vi "Define_Size_of_Array_Connected_Tracks-1.vi"(3 "[IN] Size of Longest Array\nbetween Subtracks (0,0)":i32, 4 "[IN] Indexes for Jumps":i32[](array[numeric]), 5 "[IN] Original Array Size":i32, 6 "[IN] Dot Statuses":i16[][](array[numeric])) -> (1 "[OUT] # of Eleme\nnts in new Track":i32)   [LabVIEW 2013]
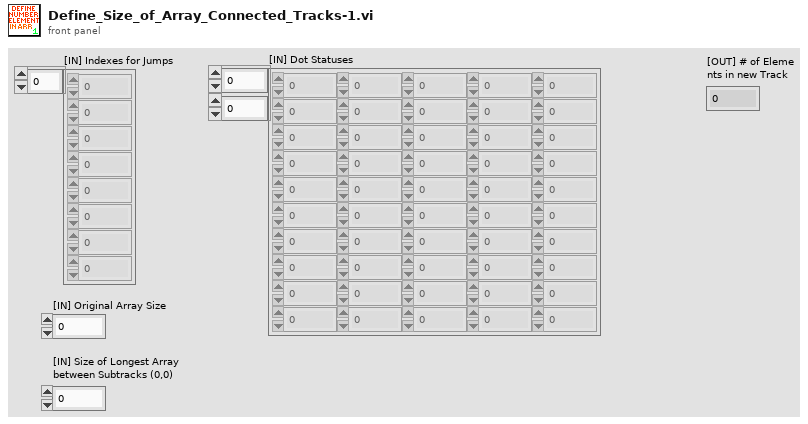
[diagram p1: front panel]
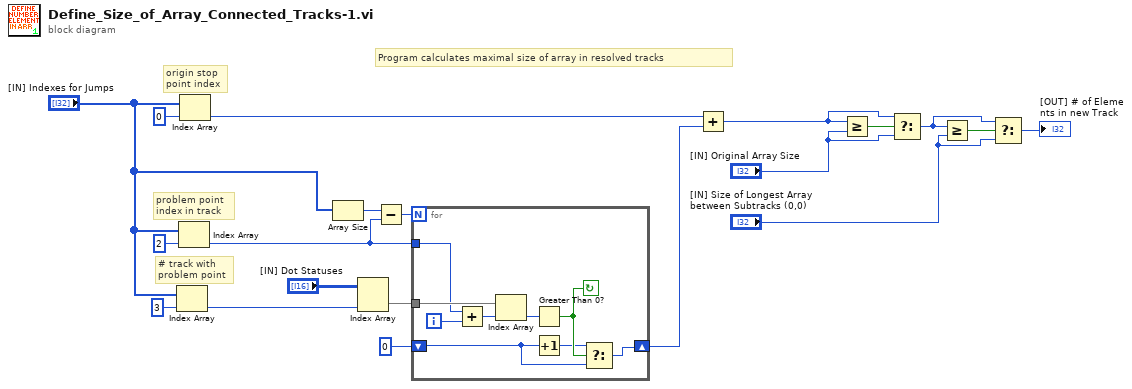
[diagram p0: block diagram]
diagram:
  # "Program calculates maximal size of array in resolved tracks"
  # "# track with \nproblem point"
  # "problem point \nindex in track"
  # "origin stop \npoint index"
  n1 = Index Array(array="[IN] Indexes for Jumps", index=3) -> (element=w16:i32)
  n2 = Index Array(array="[IN] Indexes for Jumps", index=2) -> (element=w6:i32)
  n3 = Index Array(array="[IN] Indexes for Jumps", index=0) -> (element=w7:i32)
  n4 = Array Size(array="[IN] Indexes for Jumps") -> (size(s)=w12:i32)
  n5 = Index Array(array="[IN] Dot Statuses", index (col)=w16) -> (element=w15:i16[])  [unwired: 1 in]
  n6 = Subtract(x=w12, y=w6) -> (x-y=w11:i32)
  n7 = for {
    N: w11 -> [_]
    tunnel: w15 -> [w29]
    tunnel: w6 -> [w27]
    shift-right: [w21] -> w10
    shift-left: 0 -> [w22]
    i -> [w28]
    stop <- w24 continue-if-true
    n8 = Add(x=w27, y=w28) -> (x+y=w26:i32)
    n9 = Index Array(array=w29, index=w26) -> (element=w25:i16)
    n10 = Greater Than 0?(x=w25) -> (x > 0?=w24:bool)
    n11 = Increment(x=w22) -> (x+1=w23:i32)
    n12 = Select(t=w23, s=w24, f=w22) -> (s? t:f=w21:i32)
  }
  n13 = Add(x=w7, y=w10) -> (x+y=w4:i32)
  n14 = Greater Or Equal?(x=w4, y="[IN] Original Array Size") -> (x >= y?=w9:bool)
  n15 = Select(t=w4, s=w9, f="[IN] Original Array Size") -> (s? t:f=w1:i32)
  n16 = Greater Or Equal?(x=w1, y="[IN] Size of Longest Array\nbetween Subtracks (0,0)") -> (x >= y?=w5:bool)
  n17 = Select(t=w1, s=w5, f="[IN] Size of Longest Array\nbetween Subtracks (0,0)") -> (s? t:f=→"[OUT] # of Eleme\nnts in new Track":i32)
